vi "All dates between two date.vi"(8 "To Date":timestamp format="%<%Y-%m-%d>T", 11 "From Date":timestamp format="%<%Y-%m-%d>T") -> (0 "All Days (String)":string[](array[string]), 2 "All Days":timestamp[](array[timestamp]) format="%<%Y-%m-%d>T")   [LabVIEW 2017]
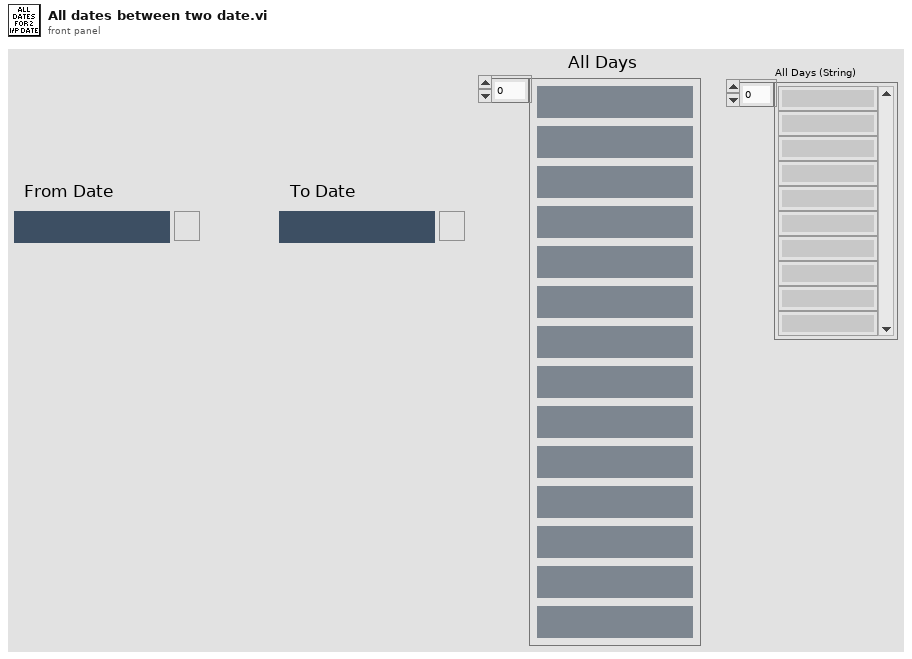
[diagram p1: front panel]
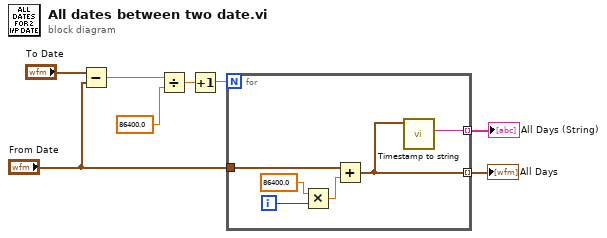
[diagram p0: block diagram]
diagram:
  n1 = Subtract(x="To Date", y="From Date") -> (x-y=w7:dbl)
  n2 = Divide(x=w7, y=86400.0) -> (x/y=w5:dbl)
  n3 = Increment(x=w5) -> (x+1=w4:dbl)
  n4 = for {
    N: w4 -> [_]
    tunnel: "From Date" -> [w11]
    tunnel: [w9] -> w2 mode=indexing
    tunnel: [w10] -> w1 mode=indexing
    i -> [w14]
    n5 = Multiply(x=86400.0 ("y"), y=w14) -> (x*y=w12:dbl)
    n6 = Add(x=w11, y=w12) -> (x+y=w9:timestamp)
    n7 = call "Timestamp to string.vi"("time stamp"=w9) -> ("Date"=w10:string)  [unwired: 8 in, 2 out]
  }
  "All Days" <- w2
  "All Days (String)" <- w1
